vi "TurboV_comm.vi"(0 "VISA resource name":refnum<visa-resource-name>="COM1", 5 "Command":T1(ring), 11 "error in (no error)":errorcluster) -> (4 "VISA resource name out":refnum<visa-resource-name>, 10 "read buffer":string, 15 "error out":errorcluster)   [LabVIEW 2015]
panel:
  out "String 2":string
  out "unsigned byte array 3":u8[](array[numeric]) format="%x"
  out "unsigned byte array":u8[](array[numeric]) format="%x"
  out "Checksum (as string)":string
  out "String":string
  out "unsigned byte array 2":u8[](array[numeric]) format="%x"
  out "return count":u32
  out "concatenated string":string
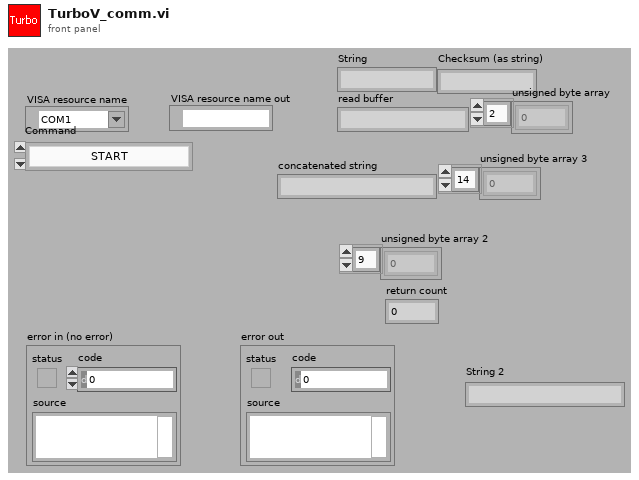
[diagram p1: front panel]
types:
  T1 = enum16{"START", "STOP", "REMOTE/SERIAL", "REMOTE", "SERIAL", "START/STOP", "PUMP STATUS", "Driving Frequency", "PUMP POWER", "PRESSURE"}
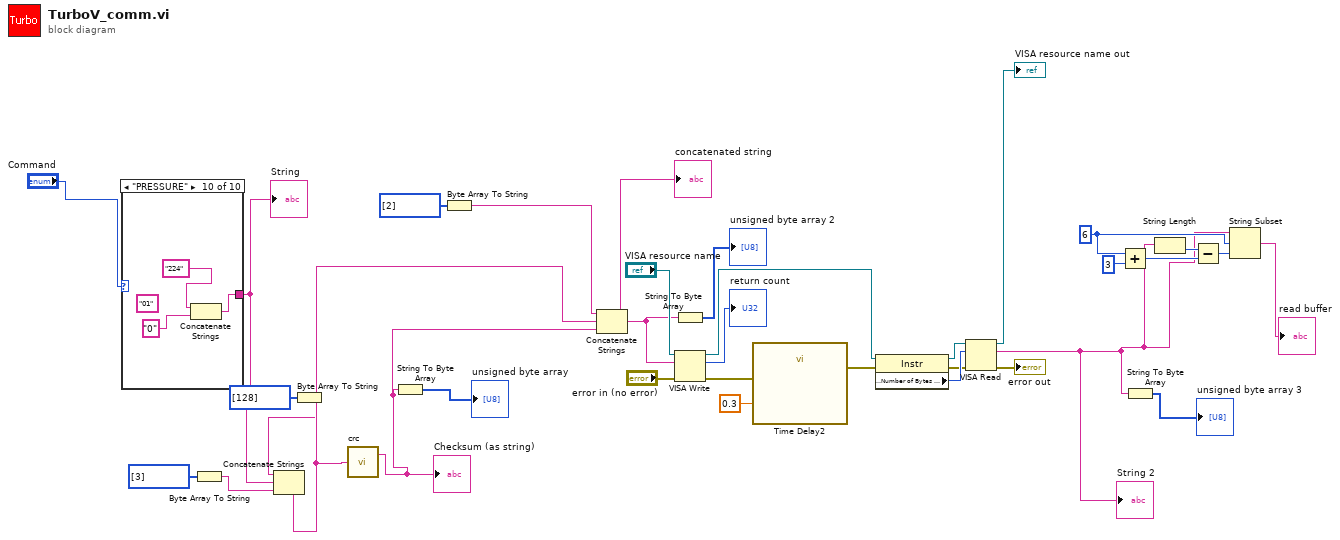
[diagram p0: block diagram]
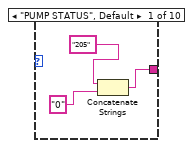
[diagram p2: hidden frame]
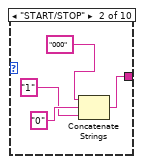
[diagram p3: hidden frame]
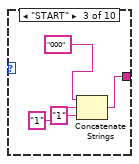
[diagram p4: hidden frame]
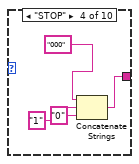
[diagram p5: hidden frame]
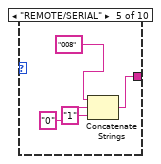
[diagram p6: hidden frame]
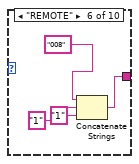
[diagram p7: hidden frame]
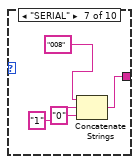
[diagram p8: hidden frame]
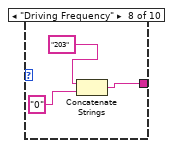
[diagram p9: hidden frame]
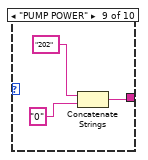
[diagram p10: hidden frame]
diagram:
  w17 = 6 ("offset (0)")
  (unwired) "01" ("string")
  n1 = case shown="\"PRESSURE\"" "Command" {
    tunnel: [w35 w38 w42 w46 w50 w54 w58 w61 w65 w67] -> w11
    frame "PUMP STATUS", Default {
      n2 = Concatenate Strings("205", "0" ("string")) -> (w35:string)
    }
    frame "START/STOP" {
      n3 = Concatenate Strings("000", "0" ("string"), "1" ("string")) -> (w38:string)
    }
    frame "START" {
      n4 = Concatenate Strings("000", "1" ("string"), "1" ("string")) -> (w42:string)
    }
    frame "STOP" {
      n5 = Concatenate Strings("000", "1" ("string"), "0" ("string")) -> (w46:string)
    }
    frame "REMOTE/SERIAL" {
      n6 = Concatenate Strings("008", "0" ("string"), "1" ("string")) -> (w50:string)
    }
    frame "REMOTE" {
      n7 = Concatenate Strings("008", "1" ("string"), "1" ("string")) -> (w54:string)
    }
    frame "SERIAL" {
      n8 = Concatenate Strings("008", "1" ("string"), "0" ("string")) -> (w58:string)
    }
    frame "Driving Frequency" {
      n9 = Concatenate Strings("203", "0" ("string")) -> (w61:string)
    }
    frame "PUMP POWER" {
      n10 = Concatenate Strings("202", "0" ("string")) -> (w65:string)
    }
    frame "PRESSURE" {
      n11 = Concatenate Strings("224", "0" ("string")) -> (w67:string)
    }
  }
  "String" <- w11
  n12 = Byte Array To String(unsigned byte array=u8[] [3]) -> (string=w10:string)
  n13 = Byte Array To String(unsigned byte array=u8[] [128]) -> (string=w6:string)
  n14 = Concatenate Strings(w6, w11, w10) -> (w9:string)
  n15 = call "crc.vi"("Input string"=w9) -> ("Checksum (as hexadecimal)"=w3:string)  [unwired: 1 out]
  "Checksum (as string)" <- w3
  n16 = String To Byte Array(string=w3) -> (unsigned byte array=→"unsigned byte array":u8[])
  n17 = Byte Array To String(unsigned byte array=u8[] [2]) -> (string=w8:string)
  n18 = Concatenate Strings(w8, w9, w3) -> (w5:string)
  "concatenated string" <- w5
  n19 = String To Byte Array(string=w5) -> (unsigned byte array=→"unsigned byte array 2":u8[])
  n20 = VISA Write(VISA resource name="VISA resource name", write buffer=w5, error in (no error)="error in (no error)") -> (VISA resource name out=w26:refnum<visa-resource-name>, return count=→"return count":u32, error out=w25:errorcluster)
  n21 = call "Time Delay2"("error in (no error)"=w25, "Delay Time (s)"=0.3) -> ("error out"=w28:errorcluster)  [unwired: 9 in]
  n22 = property class="Instr"(reference=w26, error in=w28) -> (reference out=w30:refnum<visa-resource-name>, error out=w29:errorcluster, "Serial Settings:Number of Bytes at Serial Port"=w31:u32)
  n23 = VISA Read(VISA resource name=w30, byte count=w31, error in (no error)=w29) -> (VISA resource name out=→"VISA resource name out":refnum<visa-resource-name>, read buffer=w1:string, error out=→"error out":errorcluster)  [unwired: 1 out]
  "String 2" <- w1
  n24 = Add(x=w17, y=3) -> (x+y=w15:i32)
  n25 = String To Byte Array(string=w1) -> (unsigned byte array=→"unsigned byte array 3":u8[])
  n26 = String Length(string=w1) -> (length=w19:i32)
  n27 = Subtract(x=w19, y=w15) -> (x-y=w18:i32)
  n28 = String Subset(string=w1, offset (0)=w17, length (rest)=w18) -> (substring=→"read buffer":string)
